vi "Begin.vi"(8 "error in":errorcluster) -> (0 "error out":errorcluster)   [LabVIEW 2015]
doc: "Called before other user functions, this VI is expected to open initial I/O refnums, load in file data, and do all program initialization. Notice that the <B>error out</B> terminal is simply used for data flow. Wiring it to other structures or subVIs ensures that this VI runs first."
uses:
  <vilib>/Rock Robotics/SystemInterfaces/DIO/FPGA_DIOPWMChannel.ctl
  <vilib>/Rock Robotics/WPI/Solenoid/WPI_SolenoidChannel.ctl
  <vilib>/Rock Robotics/WPI/Joystick/WPI_JoystickDeviceEnum.ctl
  <vilib>/Rock Robotics/WPI/DriverStation/WPI_DriverStationRobotMode2.ctl
  <vilib>/Rock Robotics/WPI/CAN/TalonSRX/WPI_CANTalonSRX_APIControlMode.ctl
  <vilib>/Rock Robotics/WPI/CAN/TalonSRX/WPI_CANTalonSRX_APIFeedbackSelect.ctl
  <vilib>/Rock Robotics/SystemInterfaces/spilib/spi_bus.ctl
  Robot Global Data.vi
  <vilib>/Rock Robotics/Network Tables/NT Write String Array.vi
  <vilib>/Rock Robotics/WPI/RobotDrive/WPI_RobotDriveOpen4MotorWithCANTalonSRX.vi
  <vilib>/Rock Robotics/WPI/MotorControl/WPI_MotorControlOpenCANTalonSRX.vi
  <vilib>/Rock Robotics/WPI/Solenoid/WPI_SolenoidOpenDouble.vi
  <vilib>/Rock Robotics/WPI/MotorControl/WPI_MotorControlOpen TalonSRX.vi
  ADI MXP IMU/ADI MXP IMU/FRC ADI MXP IMU.lvlib
panel:
  in  "Solenoid Lanceur Foward":T1=enum."Solenoid 1"
  in  "Right Motor Inverted":bool
  in  "Left Motor Inverted":bool=TRUE
  in  "CAN Right Slave":u8=21
  in  "CAN Left Slave":u8=11
  in  "CAN Right Master":u8=20
  in  "CAN Left Master":u8=10
  in  "Manette Co-Pilote":T2=enum."USB 1"
  in  "Manette Pilote":T2
  in  "Solenoid Lanceur Reverse":T1
  in  "PWM Pousseur":T3=enum."PWM 1"
  in  "CAN Left Shooter":u8=31
  in  "CAN Right Shooter":u8=30
  # "Lanceur"
  # "Rhino Track"
  # "Manettes"
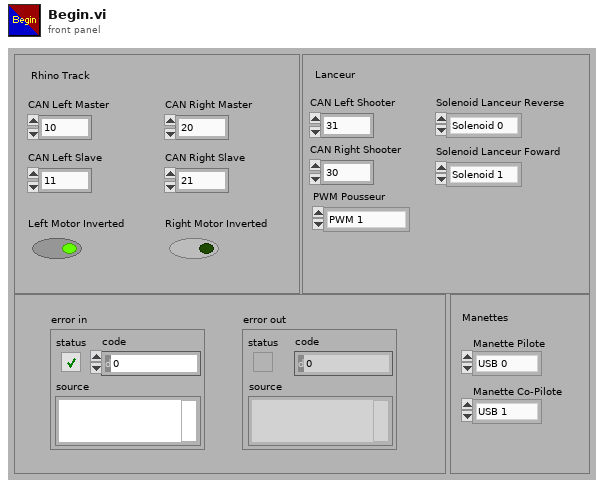
[diagram p1: front panel]
types:
  T1 = typedef "WPI_SolenoidChannel.ctl" = enum8{"Solenoid 0", "Solenoid 1", "Solenoid 2", "Solenoid 3", "Solenoid 4", "Solenoid 5", "Solenoid 6", "Solenoid 7", "Invalid"}
  T2 = typedef "WPI_JoystickDeviceEnum.ctl" = enum16{"USB 0", "USB 1", "USB 2", "USB 3", "USB 4", "USB 5"}
  T3 = typedef "FPGA_DIOPWMChannel.ctl" = enum8{"PWM 0", "PWM 1", "PWM 2", "PWM 3", "PWM 4", "PWM 5", "PWM 6", "PWM 7", "PWM 8", "PWM 9", "PWM MXP 0", "PWM MXP 1", "PWM MXP 2", "PWM MXP 3", "PWM MXP 4", "PWM MXP 5", "PWM MXP 6", "PWM MXP 7", "PWM MXP 8", "PWM MXP 9", "Invalid"}
  T4 = typedef "WPI_DriverStationRobotMode2.ctl" = enum16{"Autonomous Disabled", "Autonomous Enabled", "Teleop Disabled", "Teleop Enabled", "Disconnected", "Finish", "Test Disabled", "Test Enabled", "Emergency Stopped"}
  T5 = typedef "WPI_CANTalonSRX_APIFeedbackSelect.ctl" = enum16{"Digital Quadrature Encoder", "Analog Potentiometer", "Analog Encoder", "Count on Quad-A (Rising-Edge)", "Count on Quad-A (Falling-Edge)", "CTR Magnetic Enc (Absolute)", "CTR Magnetic Enc (Relative)", "Pulse Width"}
  T6 = typedef "WPI_CANTalonSRX_APIControlMode.ctl" = enum8{"Percent VBus", "Speed", "Position", "Slave", "Unchanged / Invalid", "Voltage Compensation", "Current", "Motion Profile"}
  T7 = typedef "WPI_RobotDriveDevRef.ctl" = cluster{"DevStatus":errorcluster, "Motors[]":T8[], "Square Inputs":bool, "Max Output":dbl}
  T8 = typedef "WPI_MotorControlDeviceRef.ctl" = cluster{"DeviceStatus":errorcluster, "Type":T9, "PWM":cluster{"PWM Channel":T3, "DeadBand":T10}, "CAN":cluster{"Device Number":u8, "Control Mode":T11, "Semaphore":T12, "Max Vout":dbl, "TalonSRX Control Mode":T6}, "Invert":bool}
  T9 = typedef "WPI_MotorControlType.ctl" = enum16{"PWM", "CAN", "CANTalonSRX"}
  T10 = typedef "WPI_PWMDeadband.ctl" = cluster{"Name":string, "maxPositivePwm":i32, "minPositivePwm":i32, "centerPwm":i32, "maxNegativePwm":i32, "minNegativePwm":i32, "angularRange":u16}
  T11 = typedef "WPI_CANJaguar_ControlMode.ctl" = enum8{"Percent VBus", "Current", "Speed", "Position", "Voltage"}
  T12 = typedef "Semaphore RefNum" = refnum<k1>
  T13 = typedef "WPI_JoystickDevRef.ctl" = cluster{"Device":T2}
  T14 = typedef "WPI_SolenoidDevRef.ctl" = cluster{"DevStatus":errorcluster, "Pneumatics Control Module":u8, "Forward Solenoid Channel":T1, "Reverse Solenoid Channel":T1}
  T15 = typedef "WPI_ServoDeviceRef.ctl" = cluster{"DeviceStatus":errorcluster, "PWM Channel":T3, "DeadBand":T10}
  T16 = typedef "spi_bus.ctl" = enum16{"SPI On-Board, CS0", "SPI On-Board, CS1", "SPI On-Board, CS2", "SPI On-Board, CS3", "SPI MXP", "Invalid"}
  T17 = typedef "FRC ADI MXP IMU.lvlib/WPI_AnalogDevicesIMUInterruptDevRef.ctl" = cluster{"SimpleGyroDevRef":T18, "InterruptRef":T19}
  T18 = typedef "FRC ADI MXP IMU.lvlib/WPI_AnalogDevicesIMUDevRef.ctl" = cluster{"DevStatus":errorcluster, "Handle":i32, "SPI Bus":T16, "Device Found":bool, "Sample Rate":dbl, "Device Ready":bool, "Yaw Axis":enum16{"X", "Y", "Z"}, "AHRS Algorithm":enum16{"Complementary", "Madgwick"}}
  T19 = typedef "WPI_InterruptRef.ctl" = cluster{"DevStatus":errorcluster, "InterruptIndex":T20}
  T20 = typedef "FPGA_InterruptIndex.ctl" = enum8{"0", "1", "2", "3", "4", "5", "6", "7", "Invalid"}
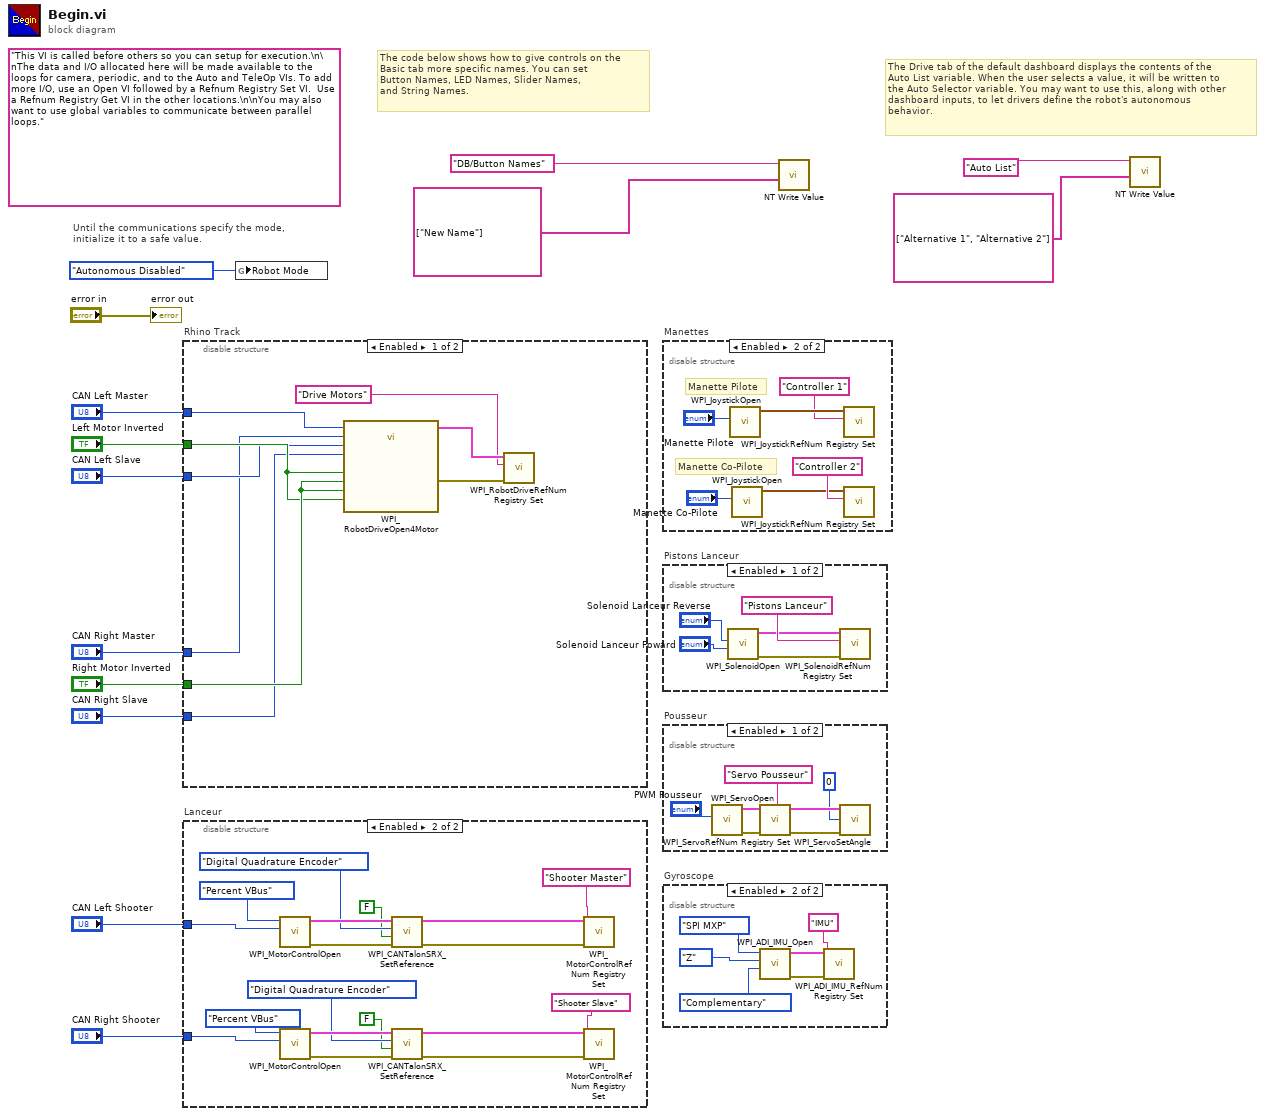
[diagram p0: block diagram]
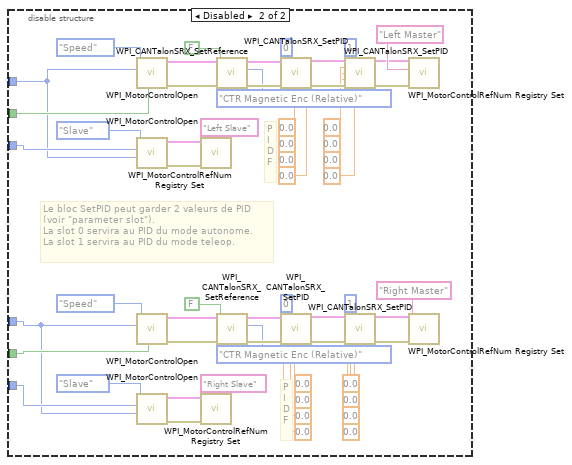
[diagram p5: hidden frame]
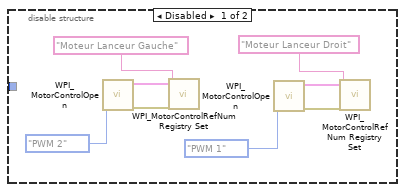
[diagram p7: hidden frame]
diagram:
  (unwired) "This VI is called before others so you can setup for execution.\n\nThe data and I/O allocated here will be made available to the loops for camera, periodic, and to the Auto and TeleOp VIs. To add more I/O, use an Open VI followed by a Refnum Registry Set VI.  Use a Refnum Registry Get VI in the other locations.\n\nYou may also want to use global variables to communicate between parallel loops."
  # "The Drive tab of the default dashboard displays the contents of the\nAuto List variable. When the user selects a value, it will be written to\nthe Auto Selector variable. You may want to use this, along with other\ndashboard inputs, to let drivers define the robot's autonomous\nbehavior."
  # "The code below shows how to give controls on the\nBasic tab more specific names. You can set\nButton Names, LED Names, Slider Names,\nand String Names."
  # "Until the communications specify the mode,\ninitialize it to a safe value."
  n1 = disable-structure "Rhino Track" shown="Enabled" {
    disable-tunnel: "Right Motor Inverted" -> [w21 w34]
    disable-tunnel: "Left Motor Inverted" -> [w20 w37]
    disable-tunnel: "CAN Right Slave" -> [w19 w33]
    disable-tunnel: "CAN Left Slave" -> [w18 w36]
    disable-tunnel: "CAN Right Master" -> [w17 w32]
    disable-tunnel: "CAN Left Master" -> [w16 w35]
    frame Enabled {
      n2 = call-poly <vilib>:"WPI_RobotDriveOpen4Motor.vi"("Rear Left Motor"=w16, "Rear Left Motor Inverted"=w20, "Rear Right Motor Inverted"=w21, "Rear Right Motor"=w17, "Front Left Motor"=w18, "Front Right Motor"=w19, "Front Left Motor Inverted"=w20, "Front Right Motor Inverted"=w21) -> ("RobotDriveDevRef"=w23:T7, "error out"=w22:errorcluster)  [unwired: 6 in]
      n3 = call <vilib>:"WPI_RobotDriveRefNum Registry Set.vi"("error in (no error)"=w22, "refnum name"="Drive Motors", "RobotDriveDevRef"=w23) -> ()  [unwired: 1 in, 8 out]
    }
    frame Disabled {
      # "Le bloc SetPID peut garder 2 valeurs de PID \n(voir \"parameter slot\").\nLa slot 0 servira au PID du mode autonome.\nLa slot 1 servira au PID du mode teleop."
      # "P\nI\nD\nF"
      # "P\nI\nD\nF"
      n4 = call-poly <vilib>:"WPI_MotorControlOpen.vi"("Invert"=w37, "Device Number"=w35, "Control Mode"=WPI_CANTalonSRX_APIControlMode."Speed") -> ("error out"=w61:errorcluster, "MotorControlDeviceRef"=w71:T8)  [unwired: 7 in]
      n5 = call-poly <vilib>:"WPI_MotorControlOpen.vi"("Master Device Number"=w35, "Device Number"=w36, "Control Mode"=WPI_CANTalonSRX_APIControlMode."Slave") -> ("error out"=w60:errorcluster, "MotorControlDeviceRef"=w79:T8)  [unwired: 7 in]
      n6 = call-poly <vilib>:"WPI_MotorControlOpen.vi"("Invert"=w34, "Device Number"=w32, "Control Mode"=WPI_CANTalonSRX_APIControlMode."Speed") -> ("error out"=w52:errorcluster, "MotorControlDeviceRef"=w70:T8)  [unwired: 7 in]
      n7 = call-poly <vilib>:"WPI_MotorControlOpen.vi"("Master Device Number"=w32, "Device Number"=w33, "Control Mode"=WPI_CANTalonSRX_APIControlMode."Slave") -> ("error out"=w59:errorcluster, "MotorControlDeviceRef"=w78:T8)  [unwired: 7 in]
      n8 = call <vilib>:"WPI_MotorControlRefNum Registry Set.vi"("error in (no error)"=w60, "refnum name"="Left Slave", "MotorControlDevRef"=w79) -> ()  [unwired: 7 in, 2 out]
      n9 = call <vilib>:"WPI_MotorControlRefNum Registry Set.vi"("error in (no error)"=w59, "refnum name"="Right Slave", "MotorControlDevRef"=w78) -> ()  [unwired: 7 in, 2 out]
      n10 = call <vilib>:"WPI_CANTalonSRX_SetReference.vi"("error in (no error)"=w61, "Reverse Feedback Sensor"=FALSE, "Feedback Reference"=WPI_CANTalonSRX_APIFeedbackSelect."CTR Magnetic Enc (Relative)", "CAN Talon SRX Ref"=w71) -> ("error out"=w68:errorcluster, "CAN Talon SRX Ref"=w69:T8)  [unwired: 6 in]
      n11 = call <vilib>:"WPI_CANTalonSRX_SetReference.vi"("error in (no error)"=w52, "Reverse Feedback Sensor"=FALSE, "Feedback Reference"=WPI_CANTalonSRX_APIFeedbackSelect."CTR Magnetic Enc (Relative)", "CAN Talon SRX Ref"=w70) -> ("error out"=w53:errorcluster, "CAN Talon SRX Ref"=w58:T8)  [unwired: 6 in]
      n12 = call <vilib>:"WPI_CANTalonSRX_SetPID.vi"("CAN Talon SRX Ref"=w69, "Parameter Slot"=u8 0, "P"=0.0, "I"=0.0, "D"=0.0, "error in (no error)"=w68, "F"=0.0) -> ("CAN Talon SRX Ref"=w67:T8, "error out"=w65:errorcluster)  [unwired: 7 in]
      n13 = call <vilib>:"WPI_CANTalonSRX_SetPID.vi"("CAN Talon SRX Ref"=w58, "Parameter Slot"=u8 0, "P"=0.0, "I"=0.0, "D"=0.0, "error in (no error)"=w53, "F"=0.0) -> ("CAN Talon SRX Ref"=w57:T8, "error out"=w54:errorcluster)  [unwired: 7 in]
      n14 = call <vilib>:"WPI_CANTalonSRX_SetPID.vi"("CAN Talon SRX Ref"=w67, "Parameter Slot"=u8 1, "P"=0.0, "I"=0.0, "D"=0.0, "error in (no error)"=w65, "F"=0.0) -> ("CAN Talon SRX Ref"=w66:T8, "error out"=w64:errorcluster)  [unwired: 7 in]
      n15 = call <vilib>:"WPI_CANTalonSRX_SetPID.vi"("CAN Talon SRX Ref"=w57, "Parameter Slot"=u8 1, "P"=0.0, "I"=0.0, "D"=0.0, "error in (no error)"=w54, "F"=0.0) -> ("CAN Talon SRX Ref"=w56:T8, "error out"=w55:errorcluster)  [unwired: 7 in]
      n16 = call <vilib>:"WPI_MotorControlRefNum Registry Set.vi"("error in (no error)"=w64, "refnum name"="Left Master", "MotorControlDevRef"=w66) -> ()  [unwired: 7 in, 2 out]
      n17 = call <vilib>:"WPI_MotorControlRefNum Registry Set.vi"("error in (no error)"=w55, "refnum name"="Right Master", "MotorControlDevRef"=w56) -> ()  [unwired: 7 in, 2 out]
    }
  }
  n18 = disable-structure "Lanceur" shown="Enabled" {
    disable-tunnel: "CAN Left Shooter" -> [_ w98]
    disable-tunnel: "CAN Right Shooter" -> [_ w97]
    frame Disabled {
      n19 = call-poly <vilib>:"WPI_MotorControlOpen.vi"("PWM Channel"=FPGA_DIOPWMChannel."PWM 2") -> ("error out"=w88:errorcluster, "MotorControlDeviceRef"=w89:T8)  [unwired: 9 in]
      n20 = call <vilib>:"WPI_MotorControlRefNum Registry Set.vi"("error in (no error)"=w88, "refnum name"="Moteur Lanceur Gauche", "MotorControlDevRef"=w89) -> ()  [unwired: 7 in, 2 out]
      n21 = call-poly <vilib>:"WPI_MotorControlOpen.vi"("PWM Channel"=FPGA_DIOPWMChannel."PWM 1") -> ("error out"=w85:errorcluster, "MotorControlDeviceRef"=w84:T8)  [unwired: 9 in]
      n22 = call <vilib>:"WPI_MotorControlRefNum Registry Set.vi"("error in (no error)"=w85, "refnum name"="Moteur Lanceur Droit", "MotorControlDevRef"=w84) -> ()  [unwired: 7 in, 2 out]
    }
    frame Enabled {
      n23 = call-poly <vilib>:"WPI_MotorControlOpen.vi"("Device Number"=w98, "Control Mode"=WPI_CANTalonSRX_APIControlMode."Percent VBus") -> ("error out"=w95:errorcluster, "MotorControlDeviceRef"=w96:T8)  [unwired: 8 in]
      n24 = call-poly <vilib>:"WPI_MotorControlOpen.vi"("Device Number"=w97, "Control Mode"=WPI_CANTalonSRX_APIControlMode."Percent VBus") -> ("error out"=w103:errorcluster, "MotorControlDeviceRef"=w104:T8)  [unwired: 8 in]
      n25 = call <vilib>:"WPI_CANTalonSRX_SetReference.vi"("error in (no error)"=w95, "Reverse Feedback Sensor"=FALSE, "Feedback Reference"=WPI_CANTalonSRX_APIFeedbackSelect."Digital Quadrature Encoder", "CAN Talon SRX Ref"=w96) -> ("error out"=w93:errorcluster, "CAN Talon SRX Ref"=w94:T8)  [unwired: 6 in]
      n26 = call <vilib>:"WPI_CANTalonSRX_SetReference.vi"("error in (no error)"=w103, "Reverse Feedback Sensor"=FALSE, "Feedback Reference"=WPI_CANTalonSRX_APIFeedbackSelect."Digital Quadrature Encoder", "CAN Talon SRX Ref"=w104) -> ("error out"=w102:errorcluster, "CAN Talon SRX Ref"=w101:T8)  [unwired: 6 in]
      n27 = call <vilib>:"WPI_MotorControlRefNum Registry Set.vi"("error in (no error)"=w93, "refnum name"="Shooter Master", "MotorControlDevRef"=w94) -> ()  [unwired: 7 in, 2 out]
      n28 = call <vilib>:"WPI_MotorControlRefNum Registry Set.vi"("error in (no error)"=w102, "refnum name"="Shooter Slave", "MotorControlDevRef"=w101) -> ()  [unwired: 7 in, 2 out]
    }
  }
  n29 = global write "Robot Global Data.vi" "Robot Mode"(WPI_DriverStationRobotMode2."Autonomous Disabled" ("Robot Mode")) -> ()
  n30 = disable-structure "Manettes" shown="Enabled" {
    frame Disabled {
    }
    frame Enabled {
      # "Manette Co-Pilote"
      # "Manette Pilote"
      n31 = call <vilib>:"WPI_JoystickOpen.vi"("JoystickDevice"="Manette Pilote") -> ("JoystickDevRef"=w109:T13)  [unwired: 10 in]
      n32 = call <vilib>:"WPI_JoystickOpen.vi"("JoystickDevice"="Manette Co-Pilote") -> ("JoystickDevRef"=w112:T13)  [unwired: 10 in]
      n33 = call <vilib>:"WPI_JoystickRefNum Registry Set.vi"("refnum name"="Controller 1", "JoystickDevRef"=w109) -> ()  [unwired: 8 in, 2 out]
      n34 = call <vilib>:"WPI_JoystickRefNum Registry Set.vi"("refnum name"="Controller 2", "JoystickDevRef"=w112) -> ()  [unwired: 8 in, 2 out]
    }
  }
  n35 = disable-structure "Pistons Lanceur" shown="Enabled" {
    frame Enabled {
      n36 = call-poly <vilib>:"WPI_SolenoidOpen.vi"("Reverse Solenoid Channel"="Solenoid Lanceur Foward", "Forward Solenoid Channel"="Solenoid Lanceur Reverse") -> ("error out"=w116:errorcluster, "SolenoidDevRef"=w115:T14)  [unwired: 8 in]
      n37 = call <vilib>:"WPI_SolenoidRefNum Registry Set.vi"("error in (no error)"=w116, "refnum name"="Pistons Lanceur", "SolenoidDevRef"=w115) -> ()  [unwired: 7 in, 2 out]
    }
    frame Disabled {
    }
  }
  n38 = disable-structure "Pousseur" shown="Enabled" {
    frame Enabled {
      n39 = call <vilib>:"WPI_ServoOpen.vi"("PWM Channel"="PWM Pousseur") -> ("error out"=w122:errorcluster, "ServoDeviceRef"=w123:T15)  [unwired: 9 in]
      n40 = call <vilib>:"WPI_ServoRefNum Registry Set.vi"("error in (no error)"=w122, "refnum name"="Servo Pousseur", "ServoDeviceRef"=w123) -> ("error out"=w119:errorcluster, "ServoDeviceRef"=w121:T15)  [unwired: 7 in]
      n41 = call <vilib>:"WPI_ServoSetAngle.vi"("error in (no error)"=w119, "Angle"=0, "ServoDeviceRef"=w121) -> ()  [unwired: 7 in, 2 out]
    }
    frame Disabled {
    }
  }
  n42 = disable-structure "Gyroscope" shown="Enabled" {
    frame Disabled {
    }
    frame Enabled {
      n43 = call "WPI_ADI_IMU_Open.vi"("AHRS Algorithm"=enum16{"Complementary", "Madgwick"}."Complementary", "Yaw Axis"=enum16{"X", "Y", "Z"}."Z", "SPI Chip Select"=spi_bus."SPI MXP") -> ("error out"=w130:errorcluster, "ADI IMU Interrupt DevRef"=w131:T17)  [unwired: 7 in]
      n44 = call "WPI_ADI_IMU_RefNum Registry Set.vi"("error in (no error)"=w130, "refnum name"="IMU", "ADI IMU Interrupt DevRef"=w131) -> ()  [unwired: 7 in, 2 out]
    }
  }
  n45 = call-poly <vilib>:"NT Write Value.vi"("String Array"=string[] ["New Name"], "Name"="DB/Button Names") -> ()  [unwired: 9 in, 1 out]
  n46 = call-poly <vilib>:"NT Write Value.vi"("String Array"=string[] ["Alternative 1", "Alternative 2"], "Name"="Auto List") -> ()  [unwired: 9 in, 1 out]
  "error out" <- "error in"
